vi "Start Connection.vi"(8 "error in (no error)":errorcluster, 11 "TCP Comm":T1) -> (0 "error out":errorcluster)   [LabVIEW 2020, in "TinyTCP.lvlib"]
uses:
  TinyTCP.lvlib
  Instance.ctl
  Ref Data.ctl
  State.ctl
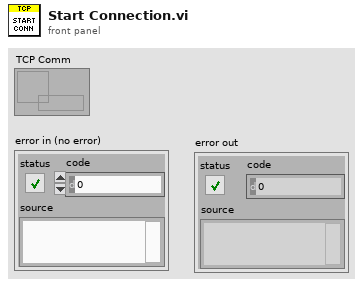
[diagram p1: front panel]
types:
  T1 = typedef "TinyTCP.lvlib/Instance.ctl" = refnum<data-value>
  T2 = typedef "TinyTCP.lvlib/Ref Data.ctl" = cluster{"TCP":refnum<k5>, "State":T3, "Server":bool, "Host":string, "Port":u16, "Listener":refnum<k5>, "Start":bool, "Disconnect":bool, "TCP Valid":bool, "TLS Enabled":bool, "Immutable TLS":refnum<k36>, "Certificate DN":string, "local-port":u16}
  T3 = typedef "TinyTCP.lvlib/State.ctl" = enum16{"Idle", "Starting", "Connecting", "Connected", "Disconnecting", "Stopped"}
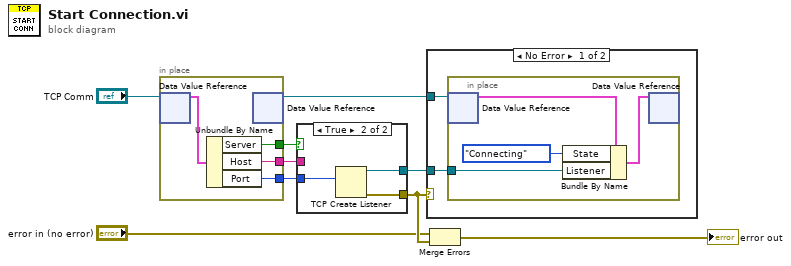
[diagram p0: block diagram]
diagram:
  n1 = in-place {
    in-place-border: [w12] -> w8
    in-place-border: [w11] -> w6
    in-place-border: [w10] -> w7
    n2 = in-place-dvr #1("TCP Comm") -> (w13:T2)  [unwired: 1 out]
    n3 = Unbundle By Name(w13) -> ("Server"=w12:bool, "Host"=w11:string, "Port"=w10:u16)
    n4 = in-place-dvr #1() -> (w5:T1)  [unwired: 1 in, 1 out]
  }
  n5 = case shown="True" w8 {
    tunnel: w7 -> [_ w16]
    tunnel: [_ w15] -> w4
    tunnel: w6 -> [_ _]
    tunnel: [_ w14] -> w3
    frame False {
    }
    frame True {
      n6 = TCP Create Listener(10:w16) -> (0:w14:errorcluster, 3:w15:refnum<k5>)  [unwired: 4 in, 1 out]
    }
  }
  n7 = case shown="No Error" w3 {
    tunnel: w5 -> [w18 _]
    tunnel: w4 -> [w17 _]
    frame No Error {
      n8 = in-place {
        in-place-border: w17 -> [w20]
        n9 = in-place-dvr #2(w18) -> (w22:T2)  [unwired: 1 out]
        n10 = Bundle By Name(cluster=w22, "State"=State."Connecting", "Listener"=w20) -> (w19:T2)
        n11 = in-place-dvr #2(w19) -> ()  [unwired: 2 out]
      }
    }
    frame Error {
    }
  }
  n12 = Merge Errors("error in (no error)", w3) -> (→"error out":errorcluster)
